vi "_tmp3.vi"() -> ()   [LabVIEW 2019]
uses:
  lib/labview_json.lvlib
panel:
  out "x = y?":bool
  out "error out":errorcluster
  out "variant":variant
  out "Variant out":variant
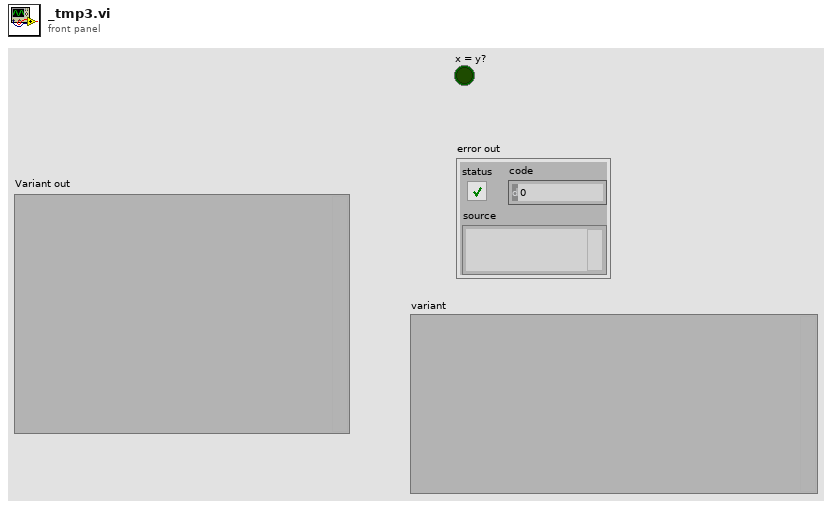
[diagram p1: front panel]
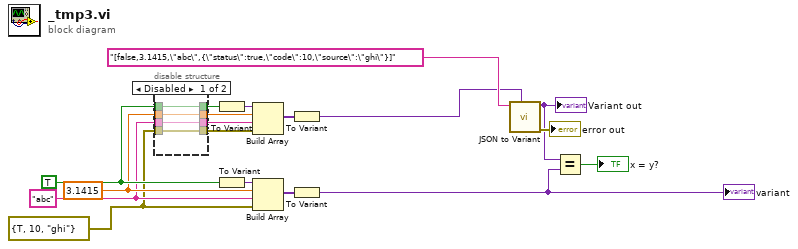
[diagram p0: block diagram]
diagram:
  w7 = errorcluster {"status"=TRUE, "code"=10, "source"="ghi"} ("error out")
  w9 = "abc"
  w11 = 3.1415
  w13 = TRUE
  n1 = disable-structure shown="Disabled" {
    disable-tunnel: w13 -> [w22 _]
    disable-tunnel: [w22 _] -> w12
    disable-tunnel: w11 -> [w21 _]
    disable-tunnel: [w21 _] -> w10
    disable-tunnel: w9 -> [w20 _]
    disable-tunnel: [w20 _] -> w8
    disable-tunnel: w7 -> [w19 _]
    disable-tunnel: [w19 _] -> w6
    frame Disabled {
    }
    frame Enabled {
    }
  }
  n2 = To Variant(anything=w12) -> (Variant=w14:variant)
  n3 = To Variant(anything=w13) -> (Variant=w17:variant)
  n4 = Build Array(w14, w10, w8, w6) -> (w15:variant[])
  n5 = Build Array(w17, w11, w9, w7) -> (w16:variant[])
  n6 = To Variant(anything=w15) -> (Variant=w5:variant)
  n7 = To Variant(anything=w16) -> (Variant=w2:variant)
  "variant" <- w2
  n8 = call "JSON to Variant.vi"("Variant Type"=w5, "JSON"="[false,3.1415,\"abc\",{\"status\":true,\"code\":10,\"source\":\"ghi\"}]") -> ("error out"=→"error out":errorcluster, "Variant out"=w3:variant)  [unwired: 8 in]
  "Variant out" <- w3
  n9 = Equal?(x=w3, y=w2) -> (x = y?=→"x = y?":bool)
